vi "increment error.vi"(8 "error in (no error)":errorcluster, 11 "MB_TCP in":refnum<class "Modbus Master CR.lvclass">) -> (0 "error out":errorcluster, 2 "N errors":i32, 3 "MB_TCP out":refnum<class "Modbus Master CR.lvclass">)   [LabVIEW 2021, in "Modbus Master CR.lvclass"]
uses:
  Modbus Master CR.lvclass
  Modbus Master CR.lvclass/Modbus Master CR.ctl
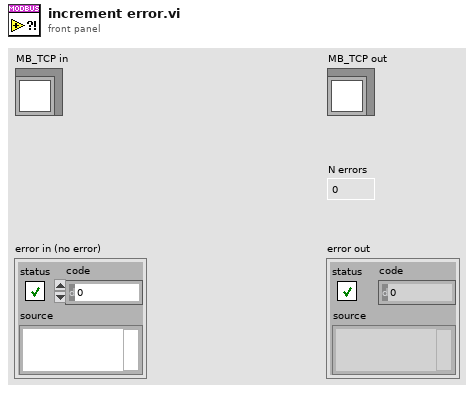
[diagram p1: front panel]
types:
  T1 = typedef "Modbus Master CR.lvclass/MB state.ctl" = cluster{"state":T2, "enable":bool, "Run":bool, "write enable":bool, "Write":bool, "connect":bool, "errors":i32}
  T2 = typedef "MB_v2.lvlib/Modbus Master CR.lvclass/MB_TCP_State.ctl" = enum8{"initialization", "redefine", "standby", "ping", "connect", "wait to reconnect", "wait to reset timeout", "configure", "requests", "close connection", "stop"}
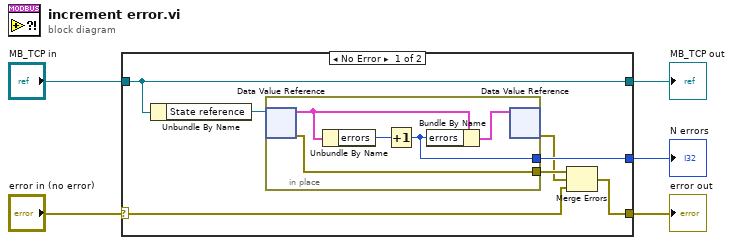
[diagram p0: block diagram]
diagram:
  n1 = case shown="No Error" "error in (no error)" {
    selector: "error in (no error)" -> [w7 w18]
    tunnel: [w6 w18] -> w1
    tunnel: [w10 w19] -> w4
    tunnel: "MB_TCP in" -> [w10 w19]
    tunnel: [w12 _] -> w2
    frame No Error {
      n2 = Unbundle By Name(w10) -> ("State reference"=w11:refnum<data-value>)
      n3 = in-place {
        in-place-border: [w14] -> w12
        in-place-border: [w13] -> w9
        n4 = in-place-dvr #1(w11) -> (w16:T1, w13:errorcluster)
        n5 = Unbundle By Name(w16) -> ("errors"=w17:i32)
        n6 = Increment(x=w17) -> (x+1=w14:i32)
        n7 = Bundle By Name(cluster=w16, "errors"=w14) -> (w15:T1)
        n8 = in-place-dvr #1(w15) -> (w8:errorcluster)  [unwired: 1 out]
      }
      n9 = Merge Errors(w9, w8, w7) -> (w6:errorcluster)
    }
    frame Error {
    }
  }
  "error out" <- w1
  "MB_TCP out" <- w4
  "N errors" <- w2
